vi "Create IMAQ Name.vi"(8 "error in (no error)":errorcluster, 10 "Name (\"\")":string, 11 "Video Frame in":refnum<class "Video Frame.lvclass">) -> (0 "error out":errorcluster, 2 "Name Out":string, 3 "Video Frame out":refnum<class "Video Frame.lvclass">)   [LabVIEW 2018, in "Video Frame.lvclass"]
uses:
  Video Frame.lvclass
  Video Frame.lvclass/Video Frame.ctl
  <resource>/objmgr/IMAQImage.rc
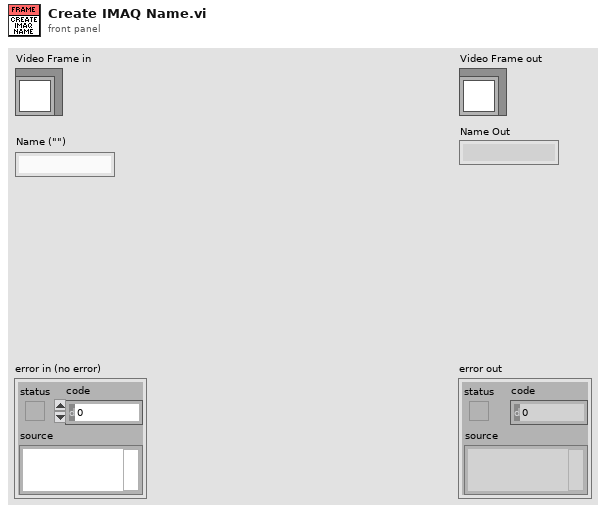
[diagram p1: front panel]
types:
  T1 = typedef "IMAQ Image.ctl" = refnum<image>
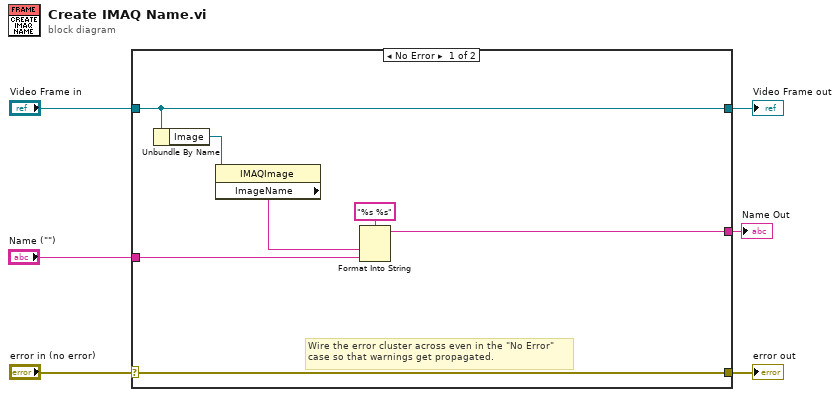
[diagram p0: block diagram]
diagram:
  n1 = case shown="No Error" "error in (no error)" {
    selector: "error in (no error)" -> [w13 w15]
    tunnel: [w13 w15] -> w5
    tunnel: [w12 w14] -> w3
    tunnel: "Video Frame in" -> [w12 w14]
    tunnel: "Name (\"\")" -> [w8 _]
    tunnel: [w7 _] -> w1
    frame No Error {
      # "Wire the error cluster across even in the \"No Error\"\ncase so that warnings get propagated."
      n2 = Unbundle By Name(w12) -> ("Image"=w11:T1)
      n3 = property class="IMAQImage"(reference=w11) -> ("ImageName"=w9:string)  [unwired: 1 in, 2 out]
      n4 = Format Into String(format string="%s %s", w9, w8) -> (resulting string=w7:string)  [unwired: 2 in, 1 out]
    }
    frame Error {
    }
  }
  "error out" <- w5
  "Video Frame out" <- w3
  "Name Out" <- w1
